vi "Scanner Configure Scan.vi"(8 "error in (no error)":errorcluster, 10 "Message Data":variant, 11 "Data Cluster in":T1={"Link"={"Connection"=enum."USB", "Host or IP address (TCP/IP)"="", "Port (Serial/USB)"="COM1"}, "VISA resource"="", "Writer Queue"=refnum, "Status"=FALSE}) -> (0 "error out":errorcluster, 3 "Data Cluster out":T1={"Link"={"Connection"=enum."USB", "Host or IP address (TCP/IP)"="", "Port (Serial/USB)"="COM1"}, "VISA resource"="", "Writer Queue"=refnum, "Status"=FALSE})   [LabVIEW 2020, in "Hiden Scanner.lvlib"]
uses:
  Hiden Scanner.lvlib
  Scanner Hardware Configuration.ctl
  support/Message Queue/Message Cluster.ctl
  support/HW Message Cluster.ctl
  <instrlib>/Hiden/Public/Scan/Scan Details.ctl
  <instrlib>/Hiden/Public/Scan/Scan Input Details.ctl
  support/Message Queue/Message Queue.lvlib
  <instrlib>/Hiden/Hiden MS.lvlib
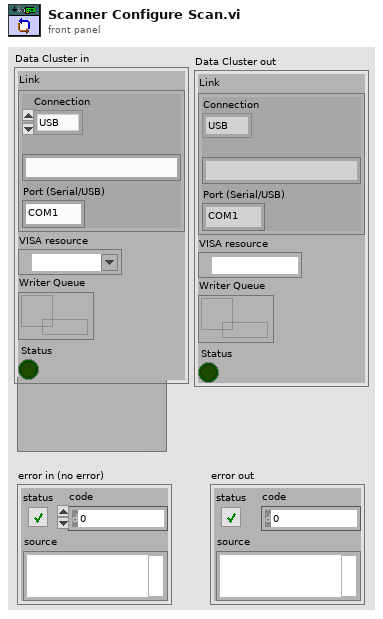
[diagram p1: front panel]
types:
  T1 = typedef "Hiden Scanner.lvlib/Scanner Hardware Configuration.ctl" = cluster{"Link":cluster{"Connection":enum16{"Serial", "TCP/IP", "USB"}, "Host or IP address (TCP/IP)":string, "Port (Serial/USB)":string}, "VISA resource":refnum<visa-resource-name>, "Writer Queue":refnum<queue>, "Status":bool}
  T2 = cluster{"Input device":string, "Autorange High":i16, "Autorange Low":i16, "Start range":i16, "Dwell (%)":u16, "Settle (%)":u16, bool, bool}
  T3 = cluster{"Device to scan":string, "Start value":dbl, "Stop value":dbl, "Increment":dbl}
  T4 = typedef "Message Queue.lvlib/HW Message Cluster.ctl" = cluster{"Writer Queue":refnum<queue>, "Writer Data":T5}
  T5 = typedef "Message Queue.lvlib/Message Cluster.ctl" = cluster{"Message":string, "Message Data":variant}
  T6 = typedef "Hiden MS.lvlib/Scan Details.ctl" = cluster{"Device to scan":string, "Start value":dbl, "Stop value":dbl, "Increment":dbl}
  T7 = typedef "Hiden MS.lvlib/Scan Input Details.ctl" = cluster{"Input device":string, "Autorange High":i16, "Autorange Low":i16, "Start range":i16, "Dwell (%)":u16, "Settle (%)":u16, "Dwell is ms?":bool, "Settle is ms?":bool}
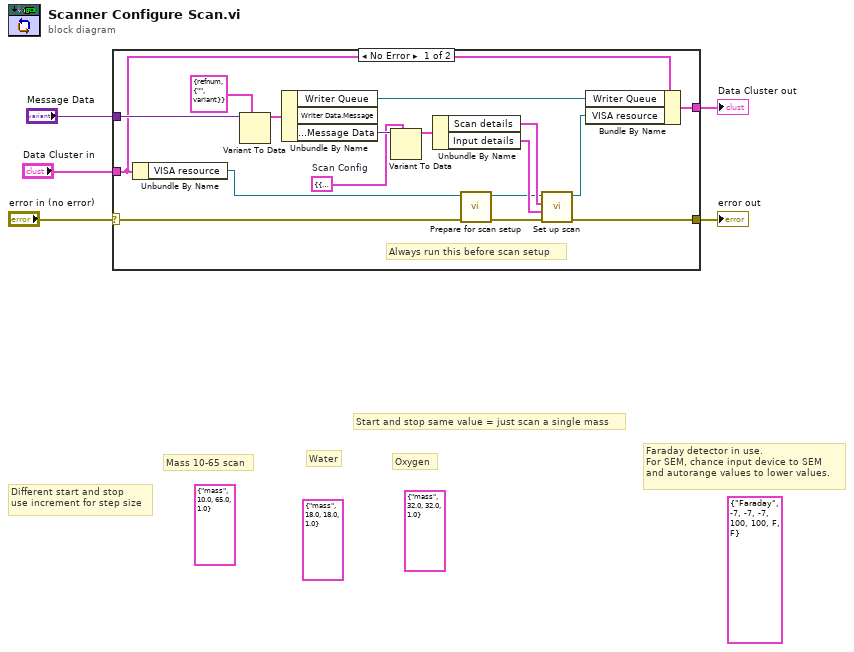
[diagram p0: block diagram]
diagram:
  (unwired) T2 {"Input device"="Faraday", "Autorange High"=-7, "Autorange Low"=-7, "Start range"=-7, "Dwell (%)"=100, "Settle (%)"=100, FALSE, FALSE} ("Input details")
  (unwired) T3 {"Device to scan"="mass", "Start value"=32.0, "Stop value"=32.0, "Increment"=1.0} ("Scan details")
  (unwired) T3 {"Device to scan"="mass", "Start value"=18.0, "Stop value"=18.0, "Increment"=1.0} ("Scan details")
  (unwired) T3 {"Device to scan"="mass", "Start value"=10.0, "Stop value"=65.0, "Increment"=1.0} ("Scan details")
  # "Faraday detector in use.\nFor SEM, chance input device to SEM\nand autorange values to lower values."
  # "Different start and stop \nuse increment for step size"
  # "Start and stop same value = just scan a single mass"
  # "Mass 10-65 scan"
  # "Oxygen"
  # "Water"
  n1 = case shown="No Error" "error in (no error)" {
    selector: "error in (no error)" -> [w6 w23]
    tunnel: "Message Data" -> [w19 _]
    tunnel: [w18 w24] -> w4
    tunnel: "Data Cluster in" -> [w16 w24]
    tunnel: [w10 w23] -> w2
    frame No Error {
      w14 = cluster{"Scan details":T6, "Input details":T7} {"Scan details"={"Device to scan"="mass", "Start value"=1.0, "Stop value"=100.0, "Increment"=1.0}, "Input details"={"Input device"="Faraday", "Autorange High"=-5, "Autorange Low"=-10, "Start range"=-7, "Dwell (%)"=100, "Settle (%)"=100, "Dwell is ms?"=FALSE, "Settle is ms?"=FALSE}}  # Scan Config
      # "Always run this before scan setup"
      n2 = Unbundle By Name(w16) -> ("VISA resource"=w9:refnum<visa-resource-name>)
      n3 = Variant To Data(type=T4 {"Writer Queue"=refnum, "Writer Data"={"Message"="", "Message Data"=variant}}, Variant=w19) -> (data=w22:T4)  [unwired: 1 in, 1 out]
      n4 = Unbundle By Name(w22) -> ("Writer Queue"=w21:refnum<queue>, "Writer Data.Message Data"=w17:variant)  [unwired: 1 out]
      n5 = Variant To Data(type=w14, Variant=w17) -> (data=w13:cluster{"Scan details":T6, "Input details":T7})  [unwired: 1 in, 1 out]
      n6 = Unbundle By Name(w13) -> ("Scan details"=w12:T6, "Input details"=w11:T7)
      n7 = call <instrlib>:"Prepare for scan setup.vi"("error in (no error)"=w6, "Connection"=w9) -> ("error out"=w7:errorcluster, "Duplicate Comms Link"=w8:refnum<visa-resource-name>)  [unwired: 8 in]
      n8 = call <instrlib>:"Set up scan.vi"("error in (no error)"=w7, "Input details"=w11, "Scan details"=w12, "Connection"=w8) -> ("error out"=w10:errorcluster, "Connection (dup)"=w15:refnum<visa-resource-name>)  [unwired: 6 in]
      n9 = Bundle By Name(cluster=w16, "Writer Queue"=w21, "VISA resource"=w15) -> (w18:T1)
    }
    frame Error {
    }
  }
  "Data Cluster out" <- w4
  "error out" <- w2
